vi "Results_plotter_Global.vi"() -> ()   [LabVIEW 2014]
panel:
  out "Full Ch Names":string[](array[string])
  in  "Plot EnFlo Tunnel Display":bool
  in  "Y plot max":dbl
  in  "Y plot min":dbl
  in  "X plot max":dbl
  in  "X plot min":dbl
  out "Filter 2 Strings":string[](array[string])
  out "Filter 1 Strings":string[](array[string])
  out "Ordinate Strings":string[](array[string])
  out "Channel names":string[](array[string])
  out "All Data":string[][](array[string])
  in  "Template":path
  in  "Series Index":i32[](array[numeric])
  out "Ordinate":i32[](array[numeric])
  out "Absisca":i32
  in  "New Values In":string[][](array[string])=[["Test data5"]]
  in  "New Chs In":string[](array[string])=["30-10-03:New:Channel new5"]
  in  "No of filter options":i32=2000
  in  "Error Bar Cluster":cluster{string[]}[](array[cluster])
  in  "Setup Filename":string
  in  "Transpose":bool
  out "Legend of ch names":string[](array[string])
  in  "Multi Ordinate?":bool
  in  "Current Data Filenames":string
  in  "Row Reference":i32[][](array[numeric])
  in  "XY Graph Cluster":cluster{dbl[], dbl[]}[](array[cluster]) {"?" format="%.2f"; "?" format="%.2f"}
  out "Plot Summary":string[][](array[string])
  out "Intensity Plot data in rows":dbl[][](array[numeric]) format="%.2f"
  out "Clear accept array":bool
  out "Legend":string[](array[string])
  out "Point info":T1(array[cluster])
  out "Plot Index values":dbl[][](array[numeric]) format="%.2f"
  in  "Value plotted Name":string
  out "Z Min":dbl format="%.2f"
  out "Z Max":dbl format="%.2f"
  in  "Surface Area":dbl format="%.2f"
  in  "Surface Integral":dbl format="%.2f"
  in  "Y Axis Name":string
  in  "X Axis Name":string
  out "Y Max":dbl format="%.2f"
  out "X Max":dbl format="%.2f"
  out "Raw Interpolation":dbl[][](array[numeric]) format="%.2f"
  in  "Y Values":dbl[](array[numeric]) format="%.2f"
  in  "X Values":dbl[](array[numeric]) format="%.2f"
  out "Y Scale":cluster{"Xo":dbl, "delta X":dbl} {"delta X" format="%.2f"; "Xo" format="%.2f"}
  out "X Scale":cluster{"Xo":dbl, "delta X":dbl} {"delta X" format="%.2f"; "Xo" format="%.2f"}
  out "Tolerances":string[](array[string])
  out "Column Header String":string
  out "Summarise":string[](array[string])
  out "Precision":string[](array[string])
  out "Dispose":string[](array[string])
  out "Description":string[](array[string])
  out "Extra Channel Values":string[](array[string])
  out "Extra Channel Names":string[](array[string])
  out "Dispose of Chs?":bool
  out "First Loop":bool
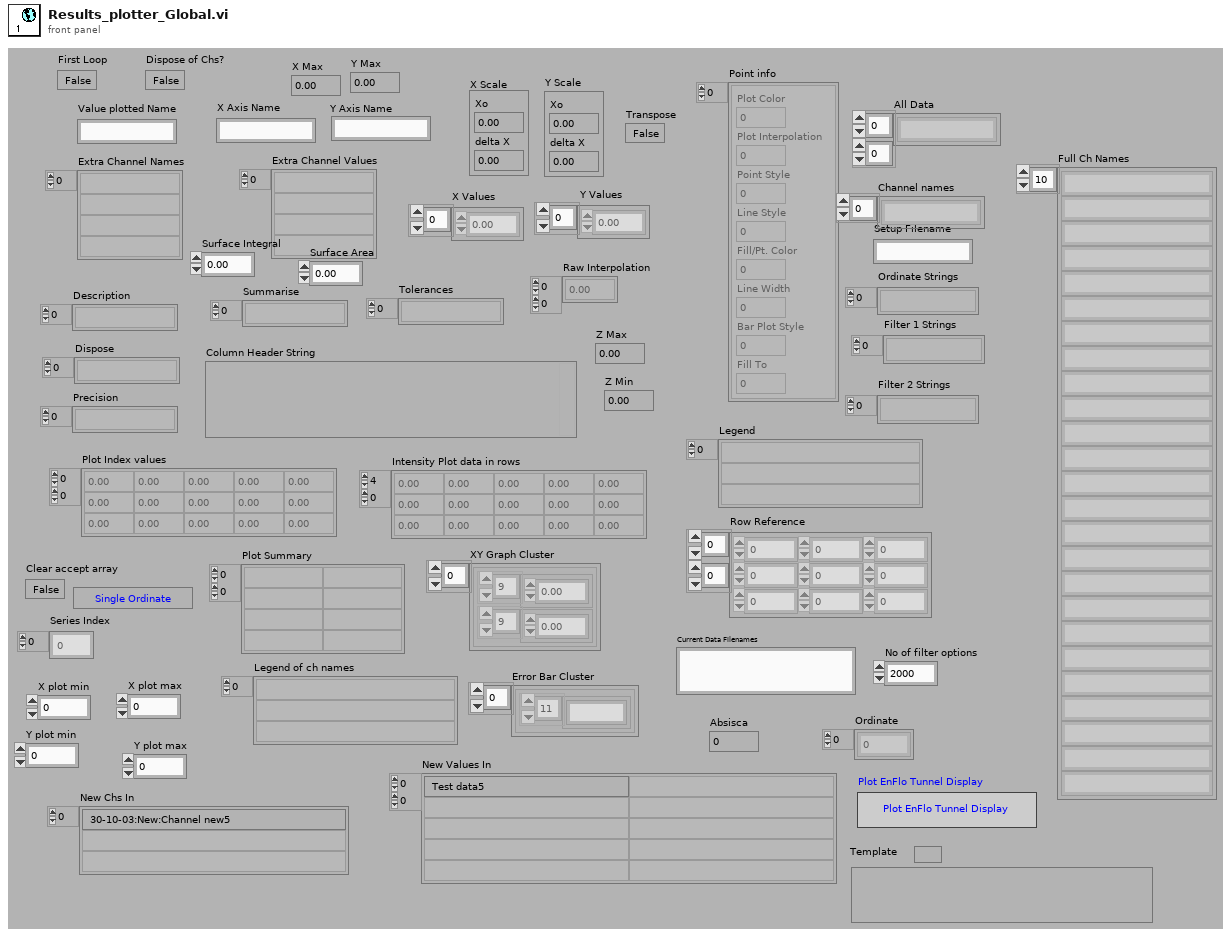
[diagram p1: front panel]
types:
  T1 = cluster{"Plot Color":u32, "Plot Interpolation":u8, "Point Style":u8, "Line Style":u8, "Fill/Pt. Color":u32, "Line Width":u8, "Bar Plot Style":u8, "Fill To":i16}[]
diagram:
